vi "ROS_Topic_Init.vi"(2 "node":string, 3 "Definitions":T1={"Topic"="/robot/head/command_head_nod", "Type"="std_msgs/Bool", "Action"=enum."Publisher", "Update (ms)"=1, "write queue"=1}) -> (1 "ROS out":T3={"topic port"=0, "Node"="", "topic"="", "type"="", "node port"=0, "error "={"status"=FALSE, "code"=0, "source"=""}, "Direction"=enum."Node", "APIs"=[], "Update (ms)"=1, "write queue"=1})   [LabVIEW 2010]
doc: "Initializes a topic and returns a ROS cluster. Required before any read or write call."
uses:
  _ROSDefinition.vi
  SubVIs/_ROSControl.ctl
  SubVIs/_ROSDirection.ctl
  Console/Servers/ServerSubs/TopicDef.ctl
panel:
  out "running?":bool
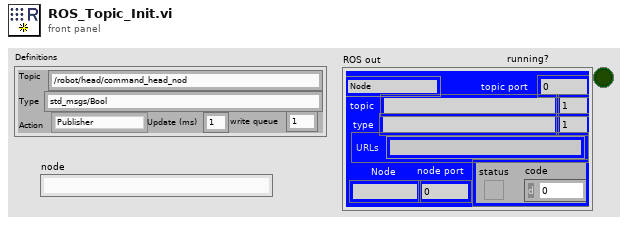
[diagram p1: front panel]
types:
  T1 = typedef "TopicDef.ctl" = cluster{"Topic":string, "Type":string, "Action":T2, "Update (ms)":u16, "write queue":u16}
  T2 = typedef "_ROSDirection.ctl" = enum16{"Node", "Publisher", "Subscriber", "Service Client"}
  T3 = typedef "_ROSControl.ctl" = cluster{"topic port":u16, "Node":string, "topic":string, "type":string, "node port":u32, "error ":errorcluster, "Direction":T2, "APIs":string[], "Update (ms)":u16, "write queue":u16}
  T4 = typedef "ServoInfo.ctl" = cluster{"vi name":string, "VI Refnum":refnum<vi>, "queue":refnum<queue>, "ROS":T3, "notifier":refnum<notifier>}
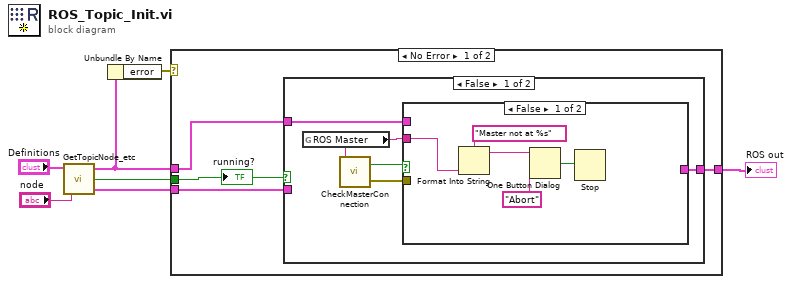
[diagram p0: block diagram]
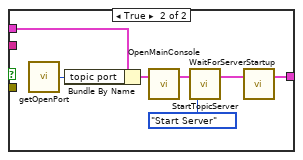
[diagram p2: hidden frame]
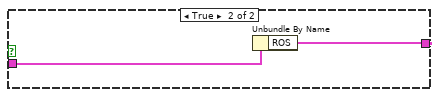
[diagram p3: hidden frame]
diagram:
  n1 = call "GetTopicNode_etc.vi"("node"="node", "Definitions"="Definitions") -> ("Server"=w1:T4, "Already running?"=w2:bool, "ROS"=w3:T3)
  n2 = Unbundle By Name(w3) -> ("error"=w4:errorcluster)
  n3 = case shown="No Error" w4 {
    tunnel: [w11 w31] -> w7
    tunnel: w3 -> [w10 w31]
    tunnel: w2 -> [w8 _]
    tunnel: w1 -> [w9 _]
    frame No Error {
      n4 = case shown="False" w8 {
        tunnel: [w15 w30] -> w11
        tunnel: w10 -> [w16 _]
        tunnel: w9 -> [_ w29]
        frame False {
          n5 = global read "_ROSDefinition.vi" "ROS Master"() -> (w13:string)
          n6 = call "CheckMasterConnection.vi"("Master IP"=w13) -> ("error out"=w12:errorcluster, "Master There?"=w14:bool)  [unwired: 1 in]
          n7 = case shown="False" w14 {
            tunnel: w16 -> [_ w26]
            tunnel: [_ w22] -> w15
            tunnel: w13 -> [w21 _]
            tunnel: w12 -> [_ _]
            frame False {
              n8 = Format Into String(format string="Master not at %s" ("message"), w21) -> (resulting string=w19:string)  [unwired: 2 in, 1 out]
              n9 = One Button Dialog(message=w19, button name ("OK")="Abort") -> (true=w17:bool)
              n10 = Stop(stop? (T)=w17) -> ()
            }
            frame True {
              n11 = call "getOpenPort.vi"() -> ("port"=w27:u16)
              n12 = Bundle By Name(cluster=w26, "topic port"=w27) -> (w25:T3)
              n13 = call "OpenMainConsole.vi"("ROS in"=w25) -> ("ROS out"=w28:T3)  [unwired: 2 in]
              n14 = call "StartTopicServer.vi"("Server Direction"=enum16{"Start Server", "Close Server"}."Start Server", "ROS in"=w28) -> ("ROS out"=w24:T3)  [unwired: 2 in]
              n15 = call "WaitForServerStartup.vi"("ROS in"=w24) -> ("ROS out"=w22:T3)  [unwired: 1 out]
            }
          }
        }
        frame True {
          n16 = Unbundle By Name(w29) -> ("ROS"=w30:T3)
        }
      }
      "running?" <- w8
    }
    frame Error {
    }
  }
  "ROS out" <- w7
